vi "Can Move To.vi"(10 "Room":string[](array[string]), 11 "Amphipod Type":string) -> (3 "Can Move To?":bool)   [LabVIEW 2019, in "23.lvlib"]
uses:
  23.lvlib
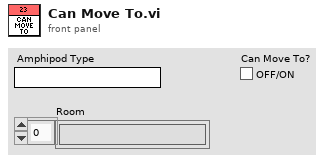
[diagram p1: front panel]
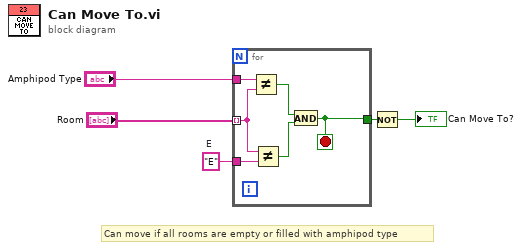
[diagram p0: block diagram]
diagram:
  w5 = "E"  # E
  # "Can move if all rooms are empty or filled with amphipod type"
  n1 = for {
    tunnel: "Room" -> [w10] mode=indexing
    tunnel: "Amphipod Type" -> [w11]
    tunnel: w5 -> [w9]
    tunnel: [w6] -> w4
    stop <- w6 stop-if-true
    n2 = Not Equal?(x=w11, y=w10) -> (x != y?=w8:bool)
    n3 = Not Equal?(x=w10, y=w9) -> (x != y?=w7:bool)
    n4 = And(x=w8, y=w7) -> (x .and. y?=w6:bool)
  }
  n5 = Not(x=w4) -> (.not. x?=→"Can Move To?":bool)
